vi "LRC.vi"(11 "Input":string) -> (3 "LRC":string)   [LabVIEW 2014]
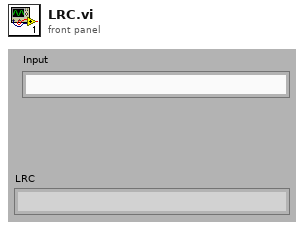
[diagram p1: front panel]
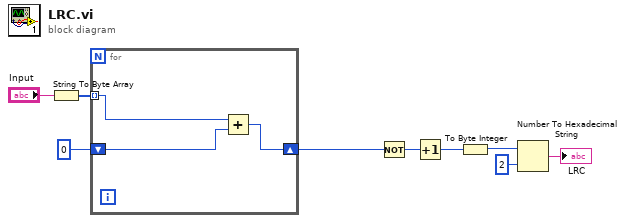
[diagram p0: block diagram]
diagram:
  n1 = String To Byte Array(string="Input") -> (unsigned byte array=w8:u8[])
  n2 = for {
    tunnel: w8 -> [w10] mode=indexing
    shift-right: [w11] -> w1
    shift-left: u8 0 -> [w12]
    n3 = Add(x=w10, y=w12) -> (x+y=w11:u8)
  }
  n4 = Not(x=w1) -> (.not. x?=w6:u8)
  n5 = Increment(x=w6) -> (x+1=w5:u8)
  n6 = To Byte Integer(number=w5) -> (8bit integer=w4:i8)
  n7 = Number To Hexadecimal String(1:i16 2 ("宽度(-)"), 2:w4) -> (0:→"LRC":string)
